vi "rgb_bueno1.vi"() -> ()   [LabVIEW 2019]
uses:
  <vilib>/Utility/file.llb/Write Delimited Spreadsheet (DBL).vi
panel:
  in  "file path (dialog if empty)":path
  out "Waveform Chart":cluster{"red":dbl, "green":dbl, "blue":dbl}(graph)
  in  "stop":bool
  out "Color":u32(colorbox)
  in  "blue":dbl(slide) scale=0.0..255.0
  in  "green":dbl(slide) scale=0.0..255.0
  in  "red":dbl(slide) scale=0.0..255.0
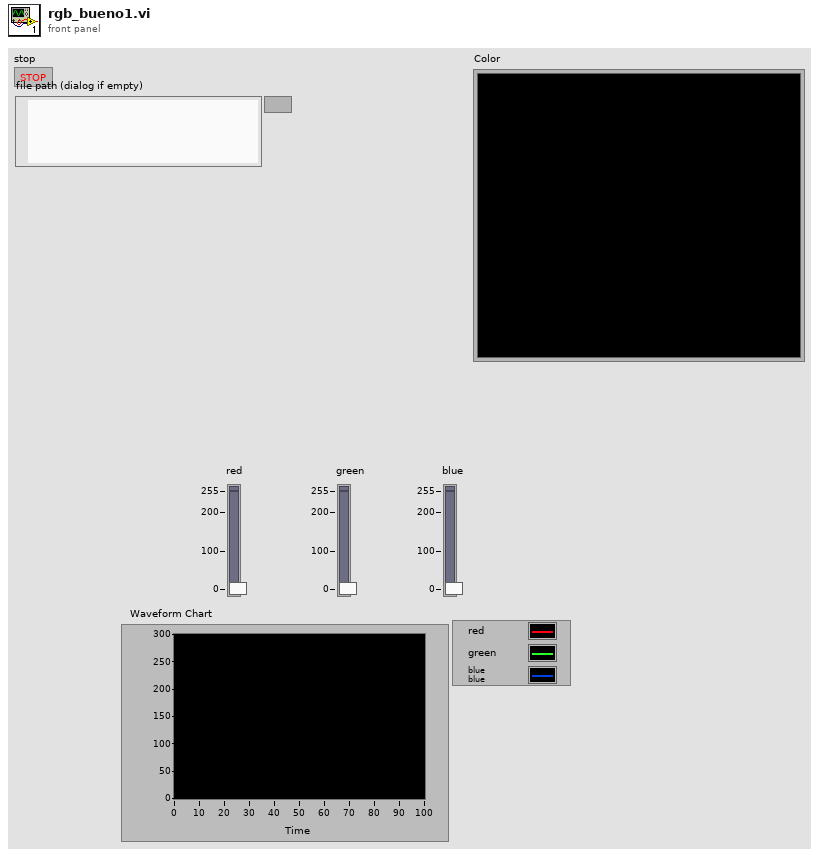
[diagram p1: front panel]
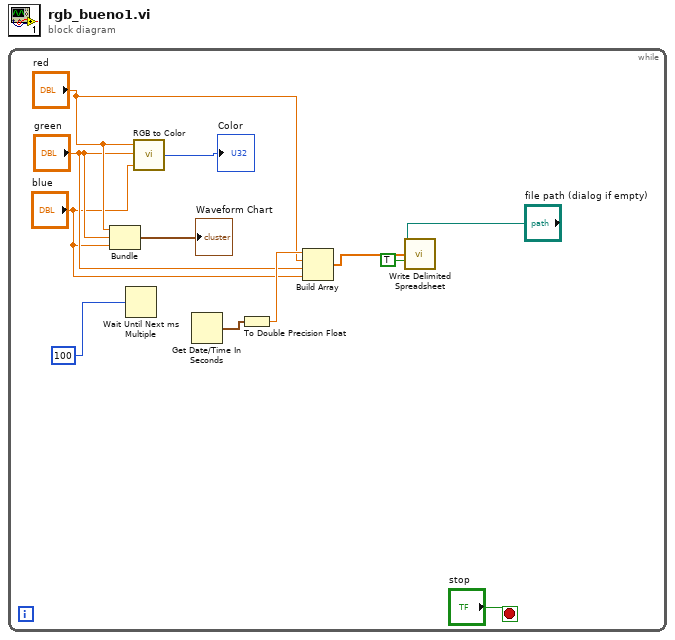
[diagram p0: block diagram]
diagram:
  n1 = while {
    stop <- "stop" stop-if-true
    n2 = Bundle("red"="red", "green"="green", "blue"="blue") -> (→"Waveform Chart":cluster{"red":dbl, "green":dbl, "blue":dbl})  [unwired: 1 in]
    n3 = Wait Until Next ms Multiple(millisecond multiple=u32 100 ("milliseconds to wait")) -> ()  [unwired: 1 out]
    n4 = call <vilib>:"RGB to Color.vi"("B"="blue", "G"="green", "R"="red") -> ("Color"=→"Color":u32)
    n5 = Get Date/Time In Seconds() -> (seconds since 1Jan1904=w8:timestamp)
    n6 = To Double Precision Float(number=w8) -> (double precision float=w7:dbl)
    n7 = Build Array(w7, "red", "green", "blue") -> (w3:dbl[])
    n8 = call-poly <vilib>:"Write Delimited Spreadsheet.vi"("file path (dialog if empty)"="file path (dialog if empty)", "1D data"=w3, "append to file? (new file:F)"=TRUE) -> ()  [unwired: 11 in, 2 out]
  }
